vi "PCO_GetTimestampMode.vi"(8 "error in (no error)":errorcluster {"code" format="%x"}, 11 "ph":u64) -> (0 "error out":errorcluster {"code" format="%x"}, 1 "wTimeStampMode":u16(ring) items=["OFF", "Binary", "Binary+ASCII", "ASCII"], 2 "ErrorMessage":i32 format="%x", 3 "ph out":u64)   [LabVIEW 2019, in "SDK.lvlib" / "RecordingControl.lvlib"]
doc: "<b>Description:</b>\nThis function returns the current timestamp mode. To obtain information about the recording time of images a timestamp can be included in the raw image data. This timestamp consists of a continuous image number and the date and time information of the camera clock. The first 14 pixels of the image data array are used to hold this information. Image numbering always starts from 1. In mode [binary] the timestamp information is packed BCD coded in the lower byte of each pixel value, so every pixel holds 2 digits of information. If the bit alignment of the camera is set to [MSB aligned] the pixel value must be shifted to the right before decoding of data can be done. In mode [ASCII] the information is written as ASCII text replacing the original image data. An 8 by 8 pixel matrix is used per ASCII digit showing white on black characters. There aIso exists mode [binary+ASCII] which is a combination of the both methods described above.\n\n<b>Format of BCD coded pixels:</b>\nPixel 1 --> Image counter(MSB) (00…99)\nPixel 2 --> Image counter (00…99)\nPixel 3 --> Image counter (00…99)\nPixel 4 --> Image counter(LSB) (00…99)\nPixel 5 --> Year (MSB) (20)\nPixel 6 --> Year (LSB) (03…99) \nPixel 7 --> Month (01..12)\nPixel 8 --> Day (01…31)\nPixel 9 --> Hour (00..23)\nPixel 10 --> Minutes (00…59)\nPixel 11 --> Seconds (00…59)\nPixel 12 --> us * 10000 (00…99)\nPixel 13 --> us * 100 (00…99)\nPixel 14 --> us (00…90)\n\n<b>Format of ASCII text:</b>\nNumber, date and time are separated by blanks\nimage number --> 8 digits [1 … 99999999]\ndate --> 9 digits [01JAN2003…31DEZ2099]\ntime --> 15 digits [00:00:00.000000…23:59:59.999990]\n\n<b>Supported camera type:</b>\nAll cameras\n\n<b>Descriptor dependency:</b>\ndwGeneralCapsDESC1: NO_TIMESTAMP"
uses:
  RecordingControl.lvlib
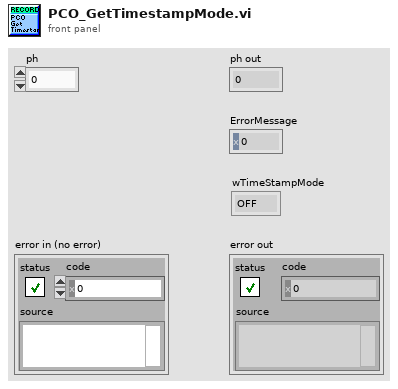
[diagram p1: front panel]
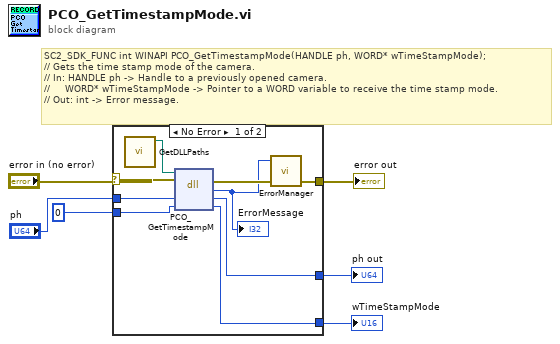
[diagram p0: block diagram]
diagram:
  # "SC2_SDK_FUNC int WINAPI PCO_GetTimestampMode(HANDLE ph, WORD* wTimeStampMode);\n// Gets the time stamp mode of the camera.\n// In: HANDLE ph -> Handle to a previously opened camera.\n//     WORD* wTimeStampMode -> Pointer to a WORD variable to receive the time stamp mode.\n// Out: int -> Error message."
  n1 = case shown="No Error" "error in (no error)" {
    selector: "error in (no error)" -> [w11 w18]
    tunnel: "ph" -> [w15 w17]
    tunnel: [w14 w17] -> w5
    tunnel: u16 0 ("wTimeStampMode") -> [w13 w16]
    tunnel: [w12 w16] -> w3
    tunnel: [w9 w18] -> w2
    frame No Error {
      n2 = call "GetDLLPaths.vi"() -> ("SC2_Cam_Path"=w7:path)  [unwired: 9 in, 2 out]
      n3 = dll-call lib="?" fn="PCO_GetTimestampMode"(path in=w7, error in=w11, "ph"=w15, "wTimeStampMode"=w13) -> (error out=w10:errorcluster, "return type"=w8:i32, "ph"=w14:u64, "wTimeStampMode"=w12:u16)  [unwired: 1 in, 1 out]
      "ErrorMessage" <- w8
      n4 = call "ErrorManager.vi"("error in (no error)"=w10, "error code"=w8) -> ("error out"=w9:errorcluster)  [unwired: 3 in]
    }
    frame Error {
    }
  }
  "ph out" <- w5
  "wTimeStampMode" <- w3
  "error out" <- w2
